vi "Periodic Tasks.vi"(8 "error in":errorcluster) -> ()   [LabVIEW 2016]
doc: "This VI runs in parallel to other tasks. It can contain as many user-defined periodic loops as you need. These can carry out PID or other sorts of timed response."
uses:
  <vilib>/Rock Robotics/SystemInterfaces/AI/FPGA_AIChannel.ctl
  <vilib>/Rock Robotics/WPI/Utilities/WPI_GetSetVariantRefNum.vi
  <vilib>/Rock Robotics/WPI/Ultrasonic/WPI_SonarMB1010AnalogOpen.vi
  <vilib>/Rock Robotics/WPI/Ultrasonic/WPI_SonarMB1010AnalogRefNum Registry Set.vi
  <vilib>/Rock Robotics/WPI/Ultrasonic/WPI_SonarMB1010AnalogGetRange.vi
  <vilib>/Rock Robotics/Network Tables/NT Write Number.vi
  <vilib>/Rock Robotics/WPI/Ultrasonic/WPI_SonarMB1010AnalogClose.vi
  <vilib>/Rock Robotics/Network Tables/NT Read Boolean.vi
  <vilib>/Rock Robotics/Network Tables/NT Write Boolean.vi
panel:
  in  "Scaling Factor":dbl=0.025
  in  "Average Bits":u8=3 max=15
  out "distance":dbl(slide)=125.0 scale=0.0..250.0 scale format="%3d"
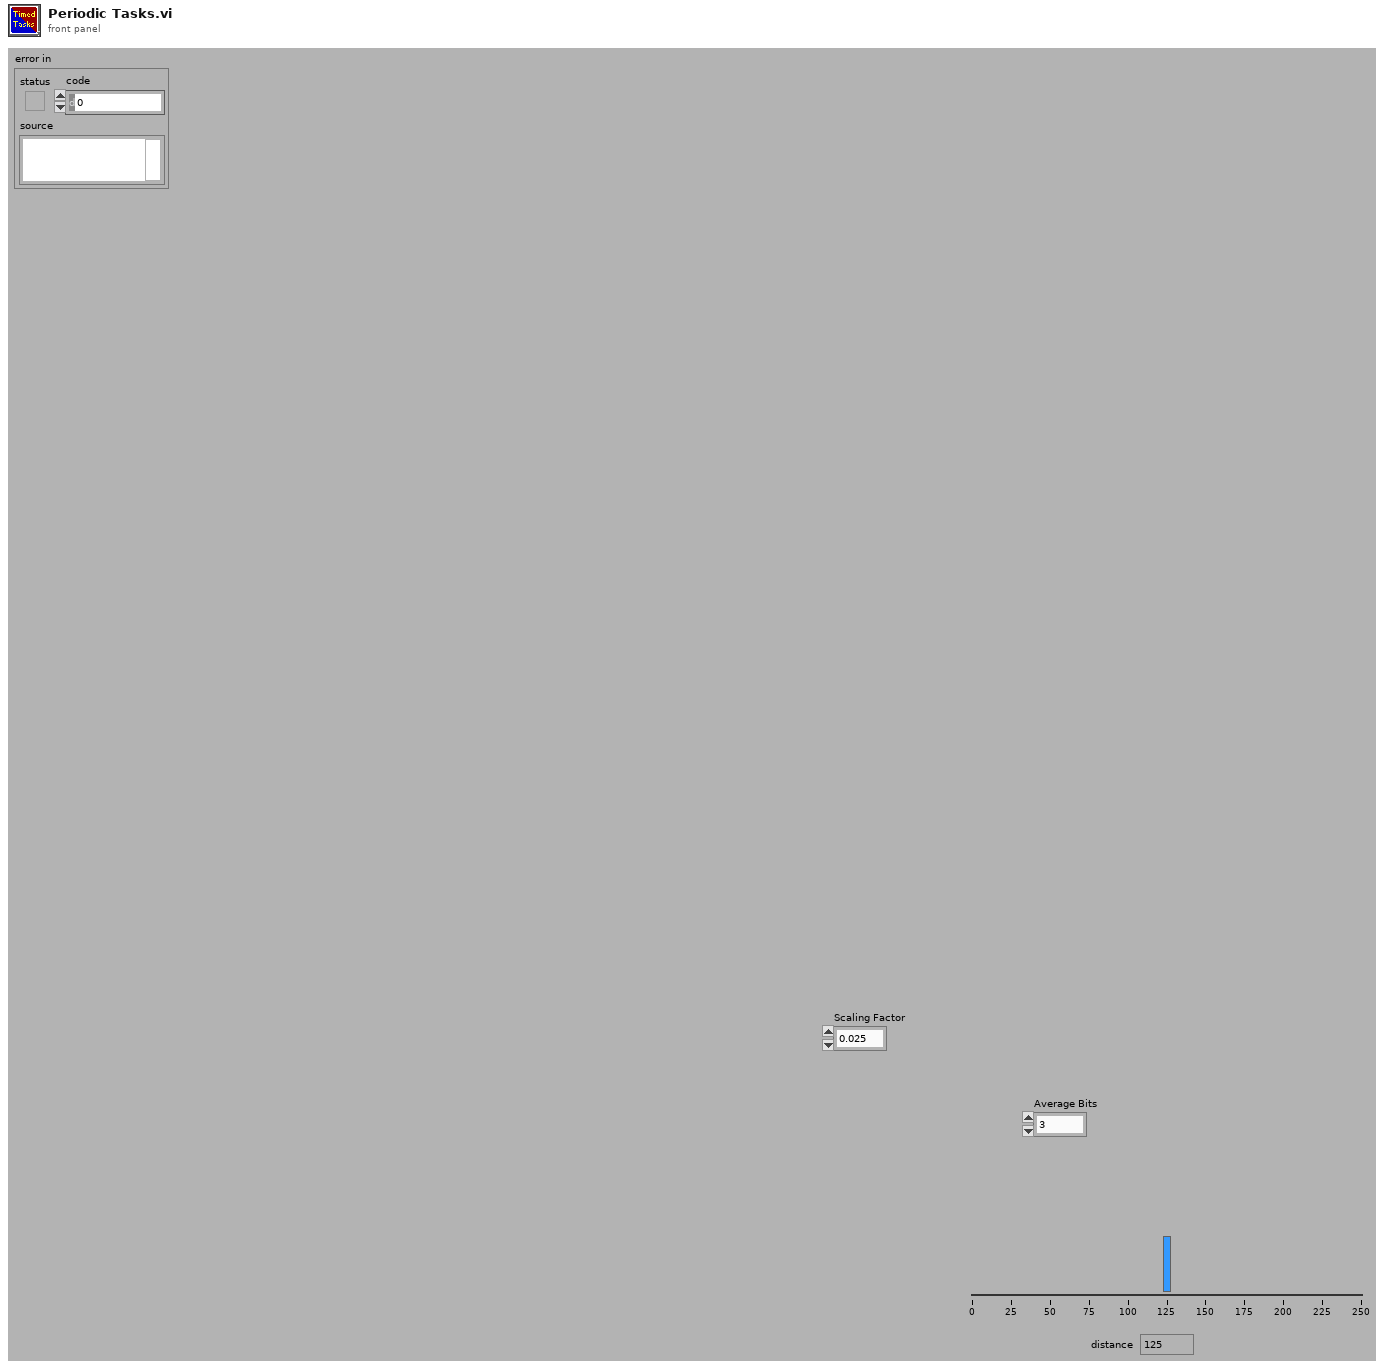
[diagram p1: front panel]
types:
  T1 = typedef "FPGA_AIChannel.ctl" = enum8{"AI 0", "AI 1", "AI 2", "AI 3", "AI MXP 0", "AI MXP 1", "AI MXP 2", "AI MXP 3", "Invalid"}
  T2 = typedef "WPI_AccelerometerDevRef.ctl" = cluster{"DevStatus":errorcluster, "Scaling":T3, "Analog Channels":T4, "I2C Bus":T5, "SPI Bus":T6, "Accel Range":T7, "ADXL Axes":T8, "Handle":i32, "Device Address":u8, "Accel Type":enum16{"Analog", "ADXL345 I2C", "ADXL345 SPI", "Internal", "ADXL362 SPI"}}
  T3 = typedef "WPI_AccelerometerScaling.ctl" = cluster{"Gain (VoltsPerG)":dbl, "Center Voltage":dbl}
  T4 = typedef "WPI_AccelerometerAnalogChannels.ctl" = cluster{"X-Axis":T1, "Y-Axis":T1, "Z-Axis":T1}
  T5 = typedef "i2c_bus.ctl" = enum16{"I2C On-Board", "I2C MXP", "Invalid"}
  T6 = typedef "spi_bus.ctl" = enum16{"SPI On-Board, CS0", "SPI On-Board, CS1", "SPI On-Board, CS2", "SPI On-Board, CS3", "SPI MXP", "Invalid"}
  T7 = typedef "ADXL345 Range.ctl" = u8
  T8 = typedef "WPI_AccelerometerADXL345 Axes.ctl" = cluster{"X-Axis":bool, "Y-Axis":bool, "Z-Axis":bool}
  T9 = typedef "WPI_GyroDevRef.ctl" = cluster{"DevStatus":errorcluster, "Analog Channel":T1, "Offset":dbl, "Gain (VoltsPerDegree/Second)":dbl, "Gyro Type":enum16{"Analog", "XRS450"}, "Handle":i32, "SPI Bus":T6, "Device Found":bool, "Sample Rate":dbl, "Calibrate On Open":bool}
  T10 = typedef "WPI_RobotDriveDevRef.ctl" = cluster{"DevStatus":errorcluster, "Motors[]":T11[], "Square Inputs":bool, "Max Output":dbl}
  T11 = typedef "WPI_MotorControlDeviceRef.ctl" = cluster{"DeviceStatus":errorcluster, "Type":T12, "PWM":cluster{"PWM Channel":T13, "DeadBand":T14}, "CAN":cluster{"Device Number":u8, "SetOutput VI Ref":variant, "GetOutput VI Ref":variant, "Enable VI Ref":variant, "Disable VI Ref":variant, "Data":variant}, "Invert":bool}
  T12 = typedef "WPI_MotorControlType.ctl" = enum16{"PWM", "CAN"}
  T13 = typedef "FPGA_DIOPWMChannel.ctl" = enum8{"PWM 0", "PWM 1", "PWM 2", "PWM 3", "PWM 4", "PWM 5", "PWM 6", "PWM 7", "PWM 8", "PWM 9", "PWM MXP 0", "PWM MXP 1", "PWM MXP 2", "PWM MXP 3", "PWM MXP 4", "PWM MXP 5", "PWM MXP 6", "PWM MXP 7", "PWM MXP 8", "PWM MXP 9", "Invalid"}
  T14 = typedef "WPI_PWMDeadband.ctl" = cluster{"Name":string, "maxPositivePwm":i32, "minPositivePwm":i32, "centerPwm":i32, "maxNegativePwm":i32, "minNegativePwm":i32, "angularRange":u16}
  T15 = typedef "WPI_JoystickDevRef.ctl" = cluster{"Device":T16}
  T16 = typedef "WPI_JoystickDeviceEnum.ctl" = enum16{"USB 0", "USB 1", "USB 2", "USB 3", "USB 4", "USB 5"}
  T17 = cluster{"JoystickDevRef":T15, "RobotDriveDevRef":T10}
  T18 = cluster{"X-Axis":dbl, "Y-Axis":dbl, "Z-Axis":dbl}
  T19 = typedef "WPI_SonarMB1010AnalogDeviceRef.ctl" = cluster{"AIDeviceRef":T20, "Scaling factor (V/in)":dbl, "Average Bits":u8}
  T20 = typedef "WPI_AnalogChannelDevRef.ctl" = cluster{"DevStatus":errorcluster, "Analog Channel":T1}
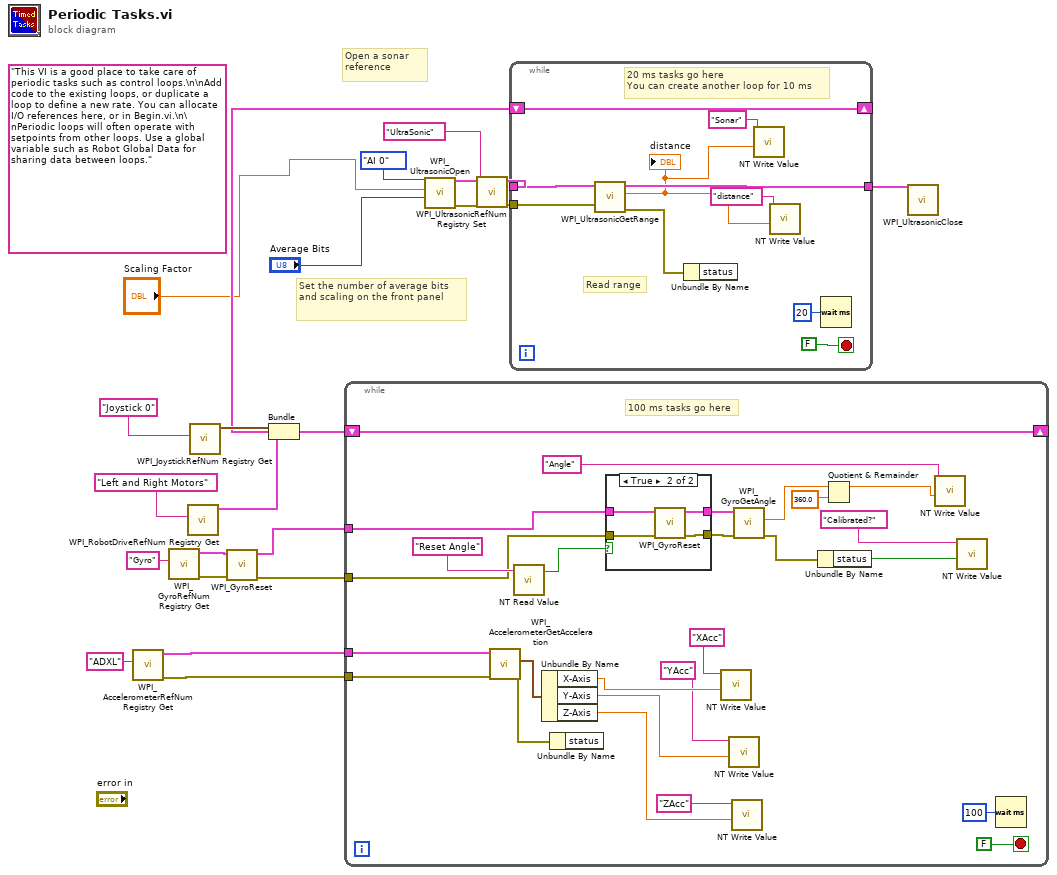
[diagram p0: block diagram]
diagram:
  (unwired) "This VI is a good place to take care of periodic tasks such as control loops.\n\nAdd code to the existing loops, or duplicate a loop to define a new rate. You can allocate I/O references here, or in Begin.vi.\n\nPeriodic loops will often operate with setpoints from other loops. Use a global variable such as Robot Global Data for sharing data between loops."
  # "Set the number of average bits and scaling on the front panel"
  # "Open a sonar reference"
  n1 = call <vilib>:"WPI_AccelerometerRefNum Registry Get.vi"("refnum name"="ADXL") -> ("error out"=w2:errorcluster, "AccelerometerDevRef"=w3:T2)  [unwired: 9 in]
  n2 = call <vilib>:"WPI_GyroRefNum Registry Get.vi"("refnum name"="Gyro") -> ("error out"=w6:errorcluster, "GyroDevRef"=w7:T9)  [unwired: 9 in]
  n3 = call <vilib>:"WPI_RobotDriveRefNum Registry Get.vi"("refnum name"="Left and Right Motors") -> ("RobotDriveDevRef"=w19:T10)  [unwired: 1 in, 9 out]
  n4 = call <vilib>:"WPI_JoystickRefNum Registry Get.vi"("refnum name"="Joystick 0") -> ("JoystickDevRef"=w20:T15)  [unwired: 1 in, 9 out]
  n5 = call <vilib>:"WPI_GyroReset.vi"("error in"=w6, "GyroDevRef"=w7) -> ("error out"=w4:errorcluster, "GyroDevRef"=w5:T9)  [unwired: 8 in]
  n6 = Bundle("JoystickDevRef"=w20, "RobotDriveDevRef"=w19) -> (w18:T17)  [unwired: 1 out]
  n7 = while {
    shift-right: [w46] -> _
    shift-left: w18 -> [w46]
    tunnel: w3 -> [w35]
    tunnel: w2 -> [w34]
    tunnel: w5 -> [w27]
    tunnel: w4 -> [w25]
    stop <- FALSE stop-if-true
    # "100 ms tasks go here"
    n8 = call <vilib>:"WPI_AccelerometerGetAcceleration.vi"("error in"=w34, "AccelerometerDevRef"=w35) -> ("error out"=w26:errorcluster, "Accelerations"=w36:T18)  [unwired: 7 in, 1 out]
    n9 = call-poly <vilib>:"NT Read Value.vi"("Name"="Reset Angle") -> ("Boolean"=w42:bool)  [unwired: 9 in, 1 out]
    n10 = Unbundle By Name(w36) -> ("X-Axis"=w33:dbl, "Y-Axis"=w32:dbl, "Z-Axis"=w31:dbl)
    n11 = Unbundle By Name(w26) -> ()  [unwired: 1 out]
    n12 = case shown="True" w42 {
      tunnel: [w50 w54] -> w38
      tunnel: w27 -> [w50 w53]
      tunnel: w25 -> [w49 w52]
      tunnel: [w49 w51] -> w24
      frame False {
      }
      frame True {
        n13 = call <vilib>:"WPI_GyroReset.vi"("error in"=w52, "GyroDevRef"=w53) -> ("error out"=w51:errorcluster, "GyroDevRef"=w54:T9)  [unwired: 8 in]
      }
    }
    n14 = call-poly <vilib>:"NT Write Value.vi"("Numeric"=w33, "Name"="XAcc") -> ()  [unwired: 9 in, 1 out]
    n15 = call-poly <vilib>:"NT Write Value.vi"("Numeric"=w32, "Name"="YAcc") -> ()  [unwired: 9 in, 1 out]
    n16 = call-poly <vilib>:"NT Write Value.vi"("Numeric"=w31, "Name"="ZAcc") -> ()  [unwired: 9 in, 1 out]
    n17 = call <vilib>:"WPI_GyroGetAngle.vi"("error in"=w24, "GyroDevRef"=w38) -> ("error out"=w23:errorcluster, "Angle"=w39:dbl)  [unwired: 5 in, 3 out]
    n18 = Unbundle By Name(w23) -> ("status"=w45:bool)
    n19 = Quotient & Remainder(x=w39, y=360.0) -> (x-y*floor(x/y)=w40:dbl)  [unwired: 1 out]
    n20 = call-poly <vilib>:"NT Write Value.vi"("Numeric"=w40, "Name"="Angle") -> ()  [unwired: 9 in, 1 out]
    n21 = call-poly <vilib>:"NT Write Value.vi"("Boolean"=w45, "Name"="Calibrated?") -> ()  [unwired: 9 in, 1 out]
    n22 = Wait (ms)(milliseconds to wait=u32 100) -> ()  [unwired: 1 out]
  }
  n23 = call-poly <vilib>:"WPI_UltrasonicOpen.vi"("Average Bits"="Average Bits", "Scaling factor (V/in)"="Scaling Factor", "Analog Channel"=FPGA_AIChannel."AI 0") -> ("error out"=w14:errorcluster, "SonarMB1010AnalogDevRef"=w12:T19)  [unwired: 7 in]
  n24 = call-poly <vilib>:"WPI_UltrasonicRefNum Registry Set.vi"("error in (no error)"=w14, "refnum name"="UltraSonic", "SonarMB1010AnalogDevRef"=w12) -> ("error out"=w10:errorcluster, "SonarMB1010AnalogDevRef"=w11:T19)  [unwired: 7 in]
  n25 = while {
    shift-right: [w62] -> _
    shift-left: w18 -> [w62]
    tunnel: [w60] -> w17
    tunnel: w11 -> [w59]
    tunnel: w10 -> [w55]
    stop <- FALSE stop-if-true
    # "Read range"
    # "20 ms tasks go here\nYou can create another loop for 10 ms"
    n26 = call-poly <vilib>:"WPI_UltrasonicGetRange.vi"("error in"=w55, "SonarMB1010AnalogDevRef"=w59) -> ("error out"=w61:errorcluster, "Distance"=w57:dbl, "SonarMB1010AnalogDevRef"=w60:T19)  [unwired: 7 in]
    "distance" <- w57
    n27 = Unbundle By Name(w61) -> ()  [unwired: 1 out]
    n28 = call-poly <vilib>:"NT Write Value.vi"("Numeric"=w57, "Name"="Sonar") -> ()  [unwired: 9 in, 1 out]
    n29 = call-poly <vilib>:"NT Write Value.vi"("Numeric"=w57, "Name"="distance") -> ()  [unwired: 9 in, 1 out]
    n30 = Wait (ms)(milliseconds to wait=u32 20) -> ()  [unwired: 1 out]
  }
  n31 = call-poly <vilib>:"WPI_UltrasonicClose.vi"("SonarMB1010AnalogDevRef"=w17) -> ()  [unwired: 10 in, 1 out]
